vi "Tree.vi"   [LabVIEW 2016, in "LV-Data.PGSQL.lvclass"]
uses:
  LV-Data.PGSQL.lvclass
  API/Read Variable (double).vi
  API/Read Variable (string).vi
  API/Read Variable (boolean).vi
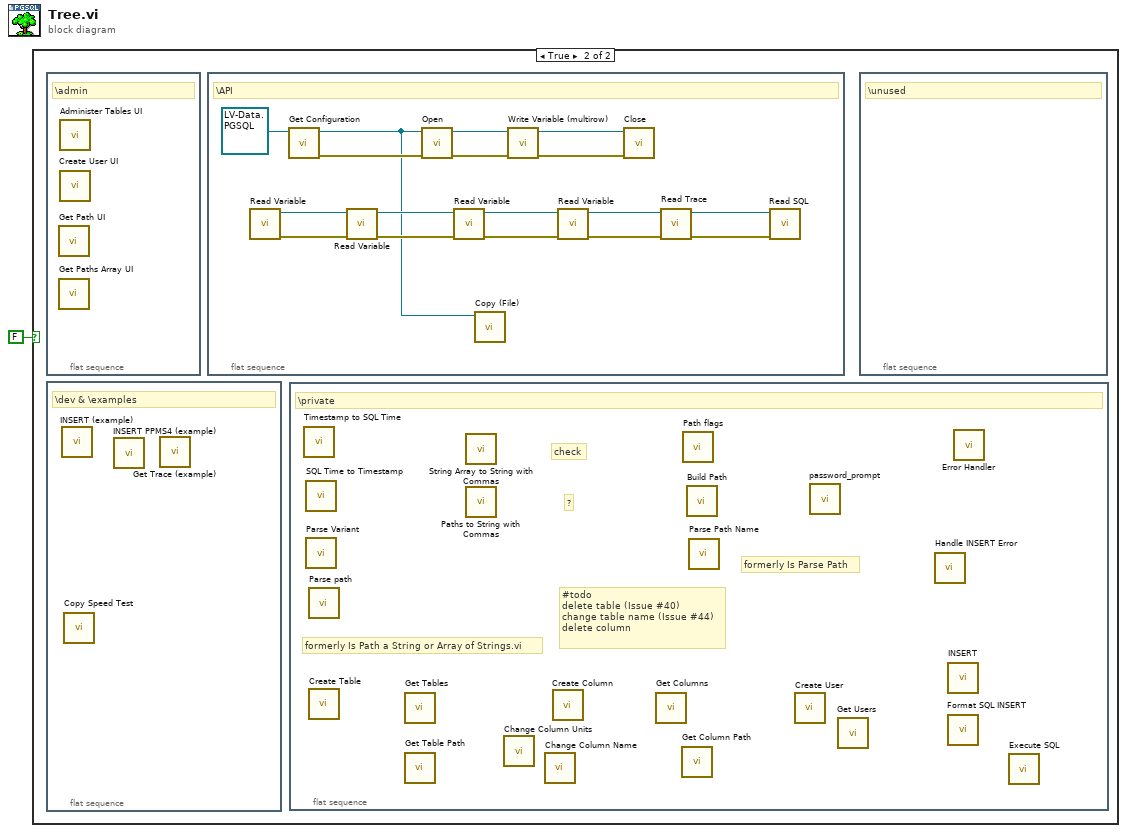
[diagram p0: block diagram]
diagram:
  n1 = case shown="True" FALSE {
    frame False {
    }
    frame True {
      n2 = flat-sequence {
        frame #0 {
          # "\\admin"
          n3 = call "Get Path UI.vi"() -> ()  [unwired: 12 in]
          n4 = call "Get Paths Array UI.vi"() -> ()  [unwired: 12 in]
          n5 = call "Administer Tables UI.vi"() -> ()  [unwired: 12 in]
          n6 = call "Create User UI.vi"() -> ()  [unwired: 12 in]
        }
      }
      n7 = flat-sequence {
        frame #0 {
          # "\\dev & \\examples"
          n8 = call "INSERT (example).vi"() -> ()  [unwired: 12 in]
          n9 = call "Copy Speed Test.vi"() -> ()  [unwired: 12 in]
          n10 = call "INSERT PPMS4 (example).vi"() -> ()  [unwired: 12 in]
          n11 = call "Get Trace (example).vi"() -> ()  [unwired: 12 in]
        }
      }
      n12 = flat-sequence {
        frame #0 {
          # "\\API"
          n13 = call-poly "Read Variable.vi"() -> ("error out"=w4:errorcluster, "Data.PGSQL out"=w3:refnum<class "LV-Data.PGSQL.lvclass">)  [unwired: 6 in, 4 out]
          n14 = call "Get Configuration.vi"("Data.PG in"=refnum<class "LV-Data.PGSQL.lvclass"> refnum) -> ("Data.PG out"=w2:refnum<class "LV-Data.PGSQL.lvclass">, "error out"=w15:errorcluster)  [unwired: 8 in]
          n15 = call-poly "Read Variable.vi"("error in (no error)"=w4, "Data.PGQL in"=w3) -> ("error out"=w9:errorcluster, "Data.PGSQL out"=w10:refnum<class "LV-Data.PGSQL.lvclass">)  [unwired: 4 in, 4 out]
          n16 = call-dynamic "Open.vi"("error in (no error)"=w15, "Data.PG in"=w2) -> ("error out"=w14:errorcluster, "Data.PG out"=w17:refnum<class "LV-Data.PGSQL.lvclass">)  [unwired: 8 in]
          n17 = call-poly "Read Variable.vi"("error in (no error)"=w9, "Data.PGQL in"=w10) -> ("error out"=w7:errorcluster, "Data.PGSQL out"=w8:refnum<class "LV-Data.PGSQL.lvclass">)  [unwired: 4 in, 4 out]
          n18 = call "Copy (File).vi"("Data.PGSQL"=w2) -> ()  [unwired: 9 in, 2 out]
          n19 = call "Write Variable (multirow).vi"("error in (no error)"=w14, "Data.PG in"=w17) -> ("error out"=w13:errorcluster, "Data.PG out"=w16:refnum<class "LV-Data.PGSQL.lvclass">)  [unwired: 7 in, 1 out]
          n20 = call-poly "Read Variable.vi"("error in (no error)"=w7, "Data.PGQL in"=w8) -> ("error out"=w5:errorcluster, "Data.PGSQL out"=w6:refnum<class "LV-Data.PGSQL.lvclass">)  [unwired: 4 in, 4 out]
          n21 = call-dynamic "Close.vi"("error in (no error)"=w13, "Data.PG in"=w16) -> ()  [unwired: 8 in, 2 out]
          n22 = call "Read Trace.vi"("error in (no error)"=w5, "Data.PGQL in"=w6) -> ("error out"=w11:errorcluster, "Data.PGSQL out"=w12:refnum<class "LV-Data.PGSQL.lvclass">)  [unwired: 5 in, 3 out]
          n23 = call "Read SQL.vi"("error in (no error)"=w11, "Data.PGQL in"=w12) -> ()  [unwired: 6 in, 4 out]
        }
      }
      n24 = flat-sequence {
        frame #0 {
          # "#todo\ndelete table (Issue #40)\nchange table name (Issue #44)\ndelete column"
          # "check"
          # "formerly Is Parse Path"
          # "?"
          # "formerly Is Path a String or Array of Strings.vi"
          # "\\private"
          n25 = call "Timestamp to SQL Time.vi"() -> ()  [unwired: 1 in, 1 out]
          n26 = call "SQL Time to Timestamp.vi"() -> ()  [unwired: 1 in, 1 out]
          n27 = call "Parse Variant.vi"() -> ()  [unwired: 7 in, 5 out]
          n28 = call "Parse path.vi"() -> ()  [unwired: 10 in, 2 out]
          n29 = call "Create Table.vi"() -> ()  [unwired: 10 in, 2 out]
          n30 = call "Get Tables.vi"() -> ()  [unwired: 8 in, 4 out]
          n31 = call "Get Table Path.vi"() -> ()  [unwired: 8 in, 4 out]
          n32 = call "String Array to String with Commas.vi"() -> ()  [unwired: 1 in, 1 out]
          n33 = call "Paths to String with Commas.vi"() -> ()  [unwired: 10 in, 2 out]
          n34 = call "Change Column Units.vi"() -> ()  [unwired: 10 in, 2 out]
          n35 = call "Change Column Name.vi"() -> ()  [unwired: 10 in, 2 out]
          n36 = call "Create Column.vi"() -> ()  [unwired: 10 in, 2 out]
          n37 = call "Get Columns.vi"() -> ()  [unwired: 7 in, 5 out]
          n38 = call "Get Column Path.vi"() -> ()  [unwired: 8 in, 4 out]
          n39 = call "Path flags.vi"() -> ()  [unwired: 11 in, 5 out]
          n40 = call "Build Path.vi"() -> ()  [unwired: 15 in, 1 out]
          n41 = call "Parse Path Name.vi"() -> ()  [unwired: 11 in, 5 out]
          n42 = call "Create User.vi"() -> ()  [unwired: 10 in, 2 out]
          n43 = call "password_prompt.vi"() -> ()  [unwired: 17 in, 3 out]
          n44 = call "Get Users.vi"() -> ()  [unwired: 9 in, 3 out]
          n45 = call "Handle INSERT Error.vi"() -> ()  [unwired: 9 in, 3 out]
          n46 = call "INSERT.vi"() -> ()  [unwired: 9 in, 3 out]
          n47 = call "Format SQL INSERT.vi"() -> ()  [unwired: 10 in, 2 out]
          n48 = call "Error Handler.vi"() -> ()  [unwired: 11 in, 1 out]
          n49 = call "Execute SQL.vi"() -> ()  [unwired: 9 in, 3 out]
        }
      }
      n50 = flat-sequence {
        frame #0 {
          # "\\unused"
        }
      }
    }
  }
